vi "扫雷.vi"() -> ()   [LabVIEW 2017]
panel:
  out "上次索引":i32
  in  "地图":u16[][](array[ring])
  out "循环计时":bool
  out "游戏进行中":bool
  out "花费时间":dbl format="%<%M:%S>T"
  out "剩余地雷数":i32
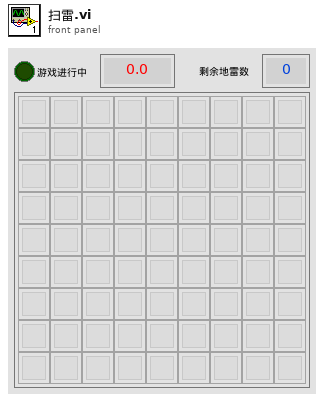
[diagram p1: front panel]
types:
  T1 = typedef "LVBoundsTypeDef.ctl" = cluster{"Width":u32, "Height":u32}
  T2 = typedef "LVPositionTypeDef.ctl" = cluster{"Left":i32, "Top":i32}
  T3 = typedef "LVPoint32TypeDef.ctl" = cluster{"Horizontal":i32, "Vertical":i32}
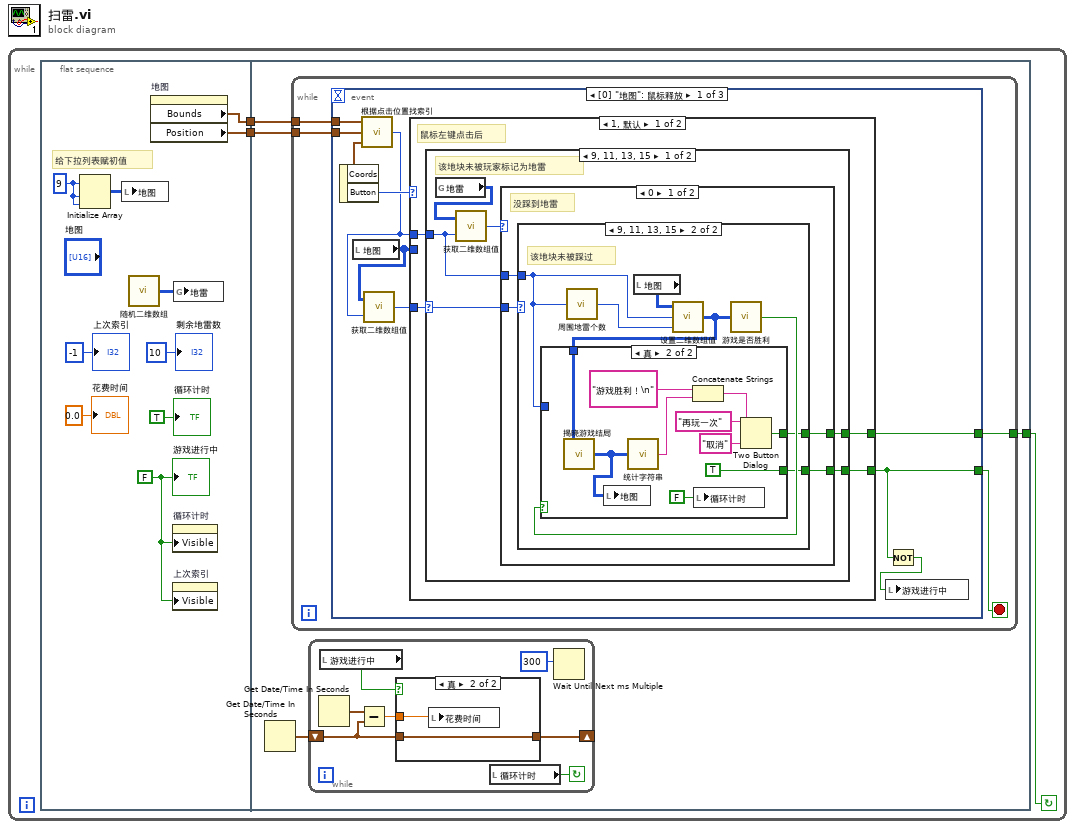
[diagram p0: block diagram]
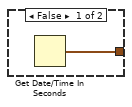
[diagram p2: hidden frame]
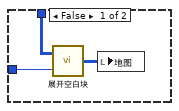
[diagram p4: hidden frame]
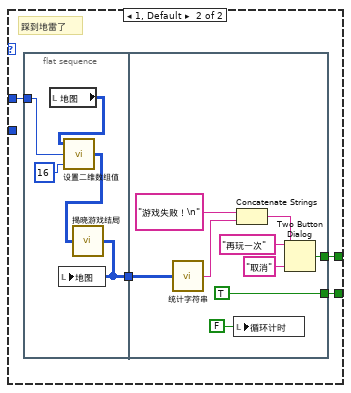
[diagram p5: hidden frame]
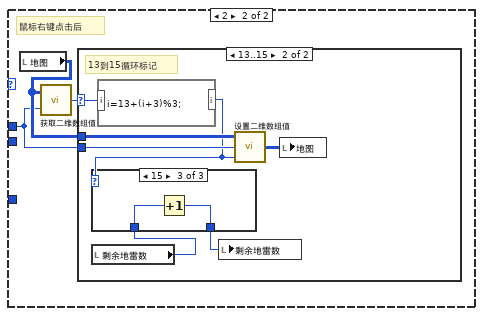
[diagram p7: hidden frame]
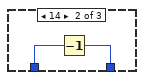
[diagram p10: hidden frame]
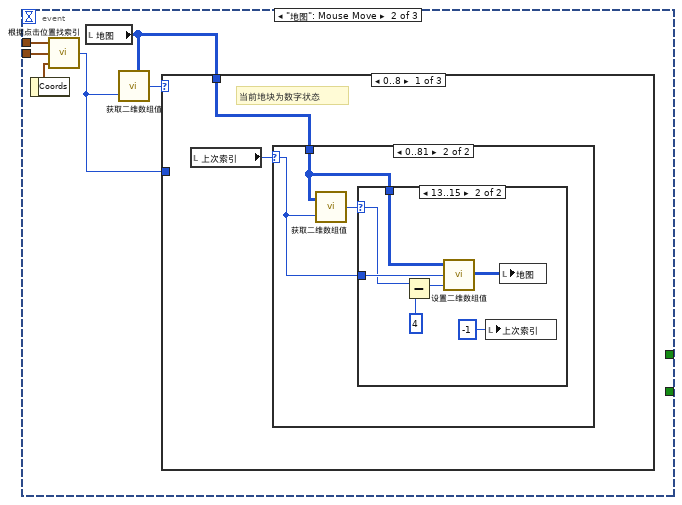
[diagram p11: hidden frame]
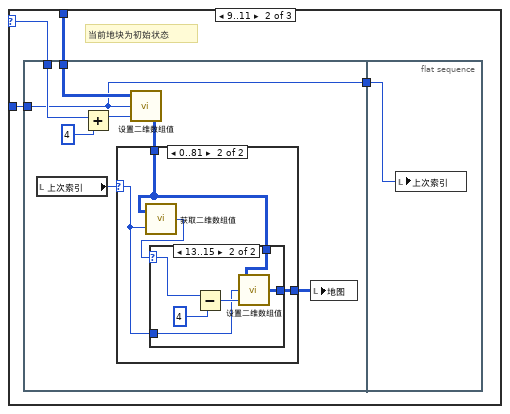
[diagram p14: hidden frame]
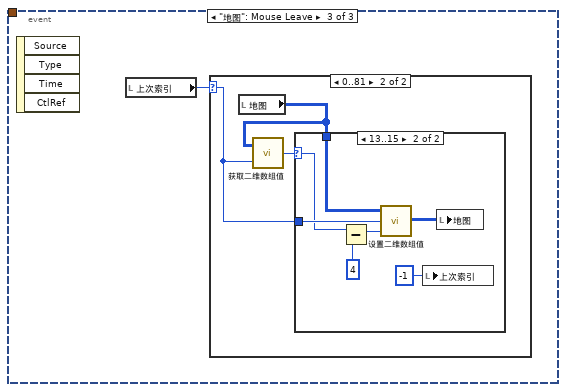
[diagram p18: hidden frame]
diagram:
  n1 = while {
    stop <- w1 continue-if-true
    n2 = flat-sequence {
      tunnel: [w6] -> w3
      tunnel: [w7] -> w2
      tunnel: [w17] -> w1
      tunnel: w3 -> [w15]
      tunnel: w2 -> [w16]
      frame #0 {
        w4 = FALSE ("游戏进行中")
        w8 = 9
        # "给下拉列表赋初值"
        n3 = Initialize Array(w8, w8, w8) -> (w9:i32[][])
        n4 = local write "地图"(w9) -> ()
        n5 = call "随机二维数组.vi"() -> ("数组"=w10:i16[][])
        n6 = property on="地图" class="Arr (严格)"() -> ("Bounds"=w7:T1, "Position"=w6:T2)  [unwired: 2 in, 2 out]
        n7 = property on="循环计时" class="Bool (严格)"("Visible"=w4) -> ()  [unwired: 2 in, 2 out]
        n8 = property on="上次索引" class="DigNum (严格)"("Visible"=w4) -> ()  [unwired: 2 in, 2 out]
        n9 = global write "全局 地雷数组.vi" "地雷"(w10) -> ()
        "剩余地雷数" <- 10 ("剩余地雷数")
        "循环计时" <- TRUE ("计时循环")
        "游戏进行中" <- w4
        "花费时间" <- 0.0 ("花费时间")
        "上次索引" <- -1 ("上次索引")
      }
      frame #1 {
        n10 = Get Date/Time In Seconds() -> (seconds since 1Jan1904=w14:timestamp)
        n11 = while {
          tunnel: [w29] -> w17
          tunnel: w16 -> [w31]
          tunnel: w15 -> [w30]
          stop <- w28 stop-if-true
          n12 = event shown="[0] \"地图\": 鼠标释放" {
            selector: _ -> [_ _ _]
            dyn-events: _ -> [_ _ _]
            timeout: _ -> [_ _ _]
            tunnel: [w37 _ _] -> w29
            tunnel: w31 -> [w41 w114 _]
            tunnel: w30 -> [w40 w113 _]
            tunnel: [w36 _ _] -> w28
            event "地图": Mouse Up {
              n13 = event-data() -> ("Coords"=w39:T3, "Button"=w38:u16)  [unwired: 1 in]
              n14 = local read "地图"() -> (w33:u16[][])
              n15 = call "根据点击位置找索引.vi"("坐标"=w39, "位置"=w40, "边界"=w41) -> ("索引"=w32:i32)
              n16 = call "获取二维数组值.vi"("索引"=w32, "数组"=w33) -> ("数值"=w34:i32)
              n17 = case shown="1, 默认" w38 {
                tunnel: [w45 _] -> w37
                tunnel: [w44 _] -> w36
                tunnel: w34 -> [w43 _]
                tunnel: w33 -> [_ _]
                tunnel: w32 -> [w42 w94]
                frame 1, Default {
                  # "鼠标左键点击后"
                  n18 = case shown="9, 11, 13, 15" w43 {
                    selector: w43 -> [w47 _]
                    tunnel: [w51 _] -> w45
                    tunnel: [w48 _] -> w44
                    tunnel: w42 -> [w46 _]
                    frame 9, 11, 13, 15 {
                      # "该地块未被玩家标记为地雷"
                      n19 = global read "全局 地雷数组.vi" "地雷"() -> (w50:i16[][])
                      n20 = call "获取二维数组值.vi"("索引"=w46, "数组"=w50) -> ("数值"=w49:i32)
                      n21 = case shown="0" w49 {
                        tunnel: [w54 w79] -> w51
                        tunnel: w47 -> [w55 _]
                        tunnel: [w53 w78] -> w48
                        tunnel: w46 -> [w52 w76]
                        frame 0 {
                          # "没踩到地雷"
                          n22 = case shown="9, 11, 13, 15" w55 {
                            tunnel: [_ w61] -> w54
                            tunnel: [_ w60] -> w53
                            tunnel: w52 -> [_ w56]
                            frame 0..8, Default {
                              # "该地块已经被踩过了"
                            }
                            frame 9, 11, 13, 15 {
                              # "该地块未被踩过"
                              n23 = call "周围地雷个数.vi"("索引"=w56) -> ("数值"=w59:i32)
                              n24 = local read "地图"() -> (w58:u16[][])
                              n25 = call "设置二维数组值.vi"("数值"=w59, "索引"=w56, "数组"=w58) -> ("输出数组"=w57:i32[][])
                              n26 = call "游戏是否胜利.vi"("地图"=w57) -> ("胜利"=w62:bool)
                              n27 = case shown="真" w62 {
                                tunnel: w57 -> [w65 w67]
                                tunnel: [_ w69] -> w61
                                tunnel: [_ TRUE] -> w60
                                tunnel: w56 -> [w63 _]
                                frame False {
                                n28 = call "展开空白块.vi"("索引"=w63, "地图"=w65) -> ("输出地图"=w64:i16[][])
                                n29 = local write "地图"(w64) -> ()
                                }
                                frame True {
                                n30 = call "揭晓游戏结局.vi"("地图"=w67) -> ("输出地图"=w66:i32[][])
                                n31 = local write "地图"(w66) -> ()
                                n32 = call "统计字符串.vi"("地图"=w66) -> ("字符串"=w71:string)
                                n33 = Concatenate Strings("游戏胜利！\n" ("消息"), w71) -> (w73:string)
                                n34 = local write "循环计时"(FALSE ("计时循环")) -> ()
                                n35 = Two Button Dialog(message=w73, 1:"取消" ("F按钮名称（“取消”）"), 2:"再玩一次" ("T按钮名称（“确定”）")) -> (T button?=w69:bool)
                                }
                              }
                            }
                          }
                        }
                        frame 1, Default {
                          # "踩到地雷了"
                          n36 = flat-sequence {
                            tunnel: [w84] -> w77
                            tunnel: w76 -> [w82]
                            tunnel: [w91] -> w79
                            tunnel: [TRUE] -> w78
                            tunnel: w77 -> [w89]
                            frame #0 {
                              n37 = local read "地图"() -> (w83:u16[][])
                              n38 = call "设置二维数组值.vi"("数值"=16, "索引"=w82, "数组"=w83) -> ("输出数组"=w80:i32[][])
                              n39 = call "揭晓游戏结局.vi"("地图"=w80) -> ("输出地图"=w84:i32[][])
                              n40 = local write "地图"(w84) -> ()
                            }
                            frame #1 {
                              n41 = call "统计字符串.vi"("地图"=w89) -> ("字符串"=w86:string)
                              n42 = local write "循环计时"(FALSE ("计时循环")) -> ()
                              n43 = Concatenate Strings("游戏失败！\n" ("消息"), w86) -> (w88:string)
                              n44 = Two Button Dialog(message=w88, 1:"取消" ("F按钮名称（“取消”）"), 2:"再玩一次" ("T按钮名称（“确定”）")) -> (T button?=w91:bool)
                            }
                          }
                        }
                      }
                    }
                    frame 10, 14, Default {
                      # "该地块被玩家标记为地雷"
                    }
                  }
                }
                frame 2 {
                  # "鼠标右键点击后"
                  n45 = local read "地图"() -> (w96:u16[][])
                  n46 = call "获取二维数组值.vi"("索引"=w94, "数组"=w96) -> ("数值"=w95:i32)
                  n47 = case shown="13..15" w95 {
                    selector: w95 -> [_ w100]
                    tunnel: w94 -> [_ w103]
                    tunnel: w96 -> [_ w102]
                    frame 0, Default {
                      # "无响应"
                    }
                    frame 13..15 {
                      # "13到15循环标记"
                      n48 = local read "剩余地雷数"() -> (w97:i32)
                      n49 = formula code="i=13+(i+3)%3;"("i"=w100) -> ("i"=w99:i32)
                      n50 = case shown="15" w99 {
                        tunnel: [w104 w105 w107] -> w98
                        tunnel: w97 -> [w104 w106 w108]
                        frame 13, Default {
                        }
                        frame 14 {
                          n51 = Decrement(x=w106) -> (x-1=w105:i32)
                        }
                        frame 15 {
                          n52 = Increment(x=w108) -> (x+1=w107:i32)
                        }
                      }
                      n53 = local write "剩余地雷数"(w98) -> ()
                      n54 = call "设置二维数组值.vi"("数值"=w99, "索引"=w103, "数组"=w102) -> ("输出数组"=w101:i32[][])
                      n55 = local write "地图"(w101) -> ()
                    }
                  }
                }
              }
              n56 = Not(x=w36) -> (.not. x?=w35:bool)
              n57 = local write "游戏进行中"(w35) -> ()
            }
            event "地图": Mouse Move {
              n58 = event-data() -> ("Coords"=w112:T3)  [unwired: 1 in]
              n59 = call "根据点击位置找索引.vi"("坐标"=w112, "位置"=w113, "边界"=w114) -> ("索引"=w109:i32)
              n60 = local read "地图"() -> (w110:u16[][])
              n61 = call "获取二维数组值.vi"("索引"=w109, "数组"=w110) -> ("数值"=w111:i32)
              n62 = case shown="0..8" w111 {
                selector: w111 -> [_ w129 _]
                tunnel: w110 -> [w115 w130 _]
                tunnel: w109 -> [_ w128 _]
                frame 0..8 {
                  # "当前地块为数字状态"
                  n63 = local read "上次索引"() -> (w116:i32)
                  n64 = case shown="0..81" w116 {
                    selector: w116 -> [_ w118]
                    tunnel: w115 -> [_ w117]
                    frame -1, Default {
                    }
                    frame 0..81 {
                      n65 = call "获取二维数组值.vi"("索引"=w118, "数组"=w117) -> ("数值"=w119:i32)
                      n66 = case shown="13..15" w119 {
                        selector: w119 -> [_ w124]
                        tunnel: w118 -> [_ w126]
                        tunnel: w117 -> [_ w125]
                        frame 0, Default {
                        }
                        frame 13..15 {
                          n67 = Subtract(x=w124, y=4) -> (x-y=w123:i32)
                          n68 = call "设置二维数组值.vi"("数值"=w123, "索引"=w126, "数组"=w125) -> ("输出数组"=w121:i32[][])
                          n69 = local write "上次索引"(-1 ("上次索引")) -> ()
                          n70 = local write "地图"(w121) -> ()
                        }
                      }
                    }
                  }
                }
                frame 9..11 {
                  # "当前地块为初始状态"
                  n71 = flat-sequence {
                    tunnel: w130 -> [w138]
                    tunnel: w129 -> [w137]
                    tunnel: w128 -> [w131]
                    tunnel: [w131] -> w127
                    tunnel: w127 -> [w151]
                    frame #0 {
                      n72 = local read "上次索引"() -> (w132:i32)
                      n73 = Add(x=w137, y=4) -> (x+y=w136:i32)
                      n74 = call "设置二维数组值.vi"("数值"=w136, "索引"=w131, "数组"=w138) -> ("输出数组"=w134:i32[][])
                      n75 = case shown="0..81" w132 {
                        selector: w132 -> [_ w142]
                        tunnel: w134 -> [w139 w143]
                        tunnel: [w139 w141] -> w133
                        frame -1, Default {
                        }
                        frame 0..81 {
                          n76 = call "获取二维数组值.vi"("索引"=w142, "数组"=w143) -> ("数值"=w140:i32)
                          n77 = case shown="13..15" w140 {
                            selector: w140 -> [_ w145]
                            tunnel: w143 -> [w144 w148]
                            tunnel: w142 -> [_ w147]
                            tunnel: [w144 w146] -> w141
                            frame 0, Default {
                            }
                            frame 13..15 {
                              n78 = Subtract(x=w145, y=4) -> (x-y=w149:i32)
                              n79 = call "设置二维数组值.vi"("数值"=w149, "索引"=w147, "数组"=w148) -> ("输出数组"=w146:i32[][])
                            }
                          }
                        }
                      }
                      n80 = local write "地图"(w133) -> ()
                    }
                    frame #1 {
                      n81 = local write "上次索引"(w151) -> ()
                    }
                  }
                }
                frame 13..15, Default {
                  # "当前地块为鼠标指定状态"
                }
              }
            }
            event "地图": Mouse Leave {
              n82 = event-data() -> ()  [unwired: 1 in, 4 out]
              n83 = local read "上次索引"() -> (w152:i32)
              n84 = case shown="0..81" w152 {
                selector: w152 -> [_ w154]
                frame -1, Default {
                }
                frame 0..81 {
                  n85 = local read "地图"() -> (w153:u16[][])
                  n86 = call "获取二维数组值.vi"("索引"=w154, "数组"=w153) -> ("数值"=w155:i32)
                  n87 = case shown="13..15" w155 {
                    selector: w155 -> [_ w160]
                    tunnel: w154 -> [_ w162]
                    tunnel: w153 -> [_ w161]
                    frame 0, Default {
                    }
                    frame 13..15 {
                      n88 = Subtract(x=w160, y=4) -> (x-y=w159:i32)
                      n89 = call "设置二维数组值.vi"("数值"=w159, "索引"=w162, "数组"=w161) -> ("输出数组"=w157:i32[][])
                      n90 = local write "上次索引"(-1 ("上次索引")) -> ()
                      n91 = local write "地图"(w157) -> ()
                    }
                  }
                }
              }
            }
          }
        }
        n92 = while {
          shift-right: [w19] -> _
          shift-left: w14 -> [w18]
          stop <- w21 continue-if-true
          n93 = Get Date/Time In Seconds() -> (seconds since 1Jan1904=w24:timestamp)
          n94 = local read "游戏进行中"() -> (w20:bool)
          n95 = Subtract(x=w24, y=w18) -> (x-y=w23:dbl)
          n96 = case shown="真" w20 {
            tunnel: w23 -> [_ w27]
            tunnel: [w25 w26] -> w19
            tunnel: w18 -> [_ w26]
            frame False {
              n97 = Get Date/Time In Seconds() -> (seconds since 1Jan1904=w25:timestamp)
            }
            frame True {
              n98 = local write "花费时间"(w27) -> ()
            }
          }
          n99 = local read "循环计时"() -> (w21:bool)
          n100 = Wait Until Next ms Multiple(millisecond multiple=300) -> ()  [unwired: 1 out]
        }
      }
    }
  }
